vi "InitActor.vi"() -> (5 "Actor":refnum<class "Actor.lvclass">)   [LabVIEW 2020, in "_Template.lvlib" / "{{Actor}}.lvlib"]
uses:
  {{Actor}}.lvlib
  jettl/jettl/Actor/Actor.lvclass
  ConcreteActor/Actor.lvclass
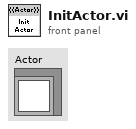
[diagram p1: front panel]
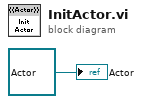
[diagram p0: block diagram]
diagram:
  "Actor" <- refnum<class "Actor.lvclass"> refnum ("_Template.lvlib:{{Actor}}.lvlib:Actor.lvclass")
